vi "Toggle Radio Buttons.vi"(8 "error in (no error)":errorcluster, 10 "Radio Buttons Refs":refnum<vi>[](array[refnum]), 11 "Activated Radio Button Ref":refnum<vi>) -> (0 "error out":errorcluster)   [LabVIEW 2020, in "hse-ui.lvlib"]
doc: "____\nHAMPEL SOFTWARE ENGINEERING v3.8.0 (2023-12-18 14:41)"
uses:
  hse-ui.lvlib
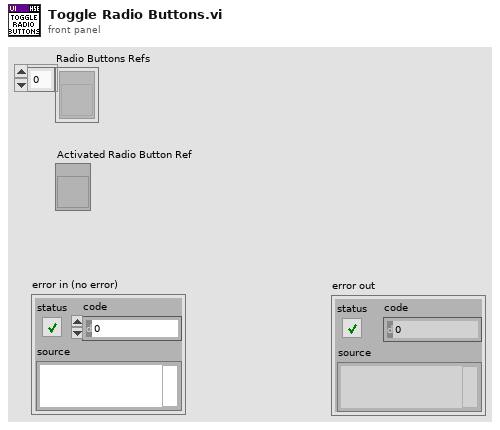
[diagram p1: front panel]
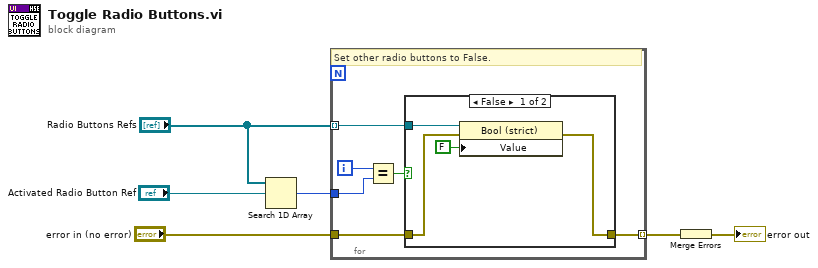
[diagram p0: block diagram]
diagram:
  n1 = Search 1D Array(1D array="Radio Buttons Refs", element="Activated Radio Button Ref") -> (index of element=w5:i32)  [unwired: 1 in]
  n2 = for {
    tunnel: "Radio Buttons Refs" -> [w10] mode=indexing
    tunnel: w5 -> [w11]
    tunnel: "error in (no error)" -> [w8]
    tunnel: [w7] -> w2 mode=indexing
    i -> [w12]
    # "Set other radio buttons to False."
    n3 = Equal?(x=w12, y=w11) -> (x = y?=w9:bool)
    n4 = case shown="False" w9 {
      tunnel: w10 -> [w16 _]
      tunnel: w8 -> [w14 w17]
      tunnel: [w13 w17] -> w7
      frame False {
        n5 = property class="Bool (strict)"(reference=w16, error in=w14, "Value"=FALSE) -> (error out=w13:errorcluster)  [unwired: 1 out]
      }
      frame True {
      }
    }
  }
  n6 = Merge Errors(w2) -> (→"error out":errorcluster)
